vi "Run 04.vi"(11 "NXT/EV3 in":T1) -> (3 "EV3 out":T1)   [LabVIEW 2016]
uses:
  <vilib>/NXT/Subs/LVHSConnector.ctl
  <vilib>/NXT/LegoClasses/BrickReference/BrickReference.lvclass
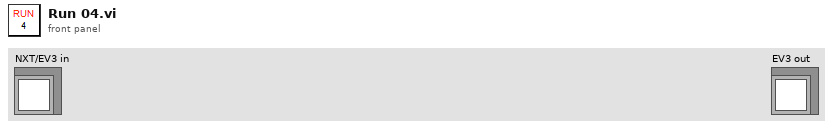
[diagram p1: front panel]
types:
  T1 = typedef "LVHSConnector.ctl" = refnum<class "BrickReference.lvclass">
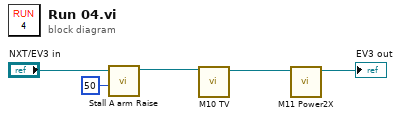
[diagram p0: block diagram]
diagram:
  n1 = call "Stall A arm Raise.vi"("Power"=i8 50, "NXT/EV3"="NXT/EV3 in") -> ("NXT/EV3"=w1:T1)  [unwired: 9 in]
  n2 = call "M10 TV.vi"("NXT/EV3"=w1) -> ("EV3 out"=w5:T1)  [unwired: 10 in]
  n3 = call "M11 Power2X.vi"("NXT/EV3"=w5) -> ("EV3 out"=→"EV3 out":T1)  [unwired: 10 in]
